vi "S7COMM - Siemens Date & Time to Timestamp.vi"(8 "error in (no error)":errorcluster, 11 "S7 DATE_AND_TIME":u8[](array[numeric])) -> (0 "error out":errorcluster, 1 "Invalid Timestamp":bool, 2 "DT":T1 {"Weekday" items=["Sunday"=1, "Monday"=2, "Tuesday"=3, "Wednesday"=4, "Thursday"=5, "Friday"=6, "Saturday"=7]; "Month" items=["Jan"=1, "Feb"=2, "Mar"=3, "Apr"=4, "May"=5, "Jun"=6, "Jul"=7, "Aug"=8, "Sep"=9, "Oct"=10, "Nov"=11, "Dec"=12]}, 3 "Time Stamp":timestamp)   [LabVIEW 2014, in "S7NetCom.lvclass"]
uses:
  S7NetCom.lvclass
  S7COMM - DTL--cluster.ctl
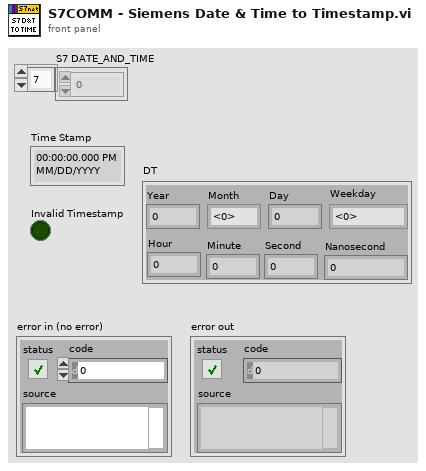
[diagram p1: front panel]
types:
  T1 = typedef "S7NetCom.lvclass/S7COMM - DTL--cluster.ctl" = cluster{"Year":u16, "Month":u8, "Day":u8, "Hour":u8, "Minute":u8, "Second":u8, "Nanosecond":u32, "Weekday":u8}
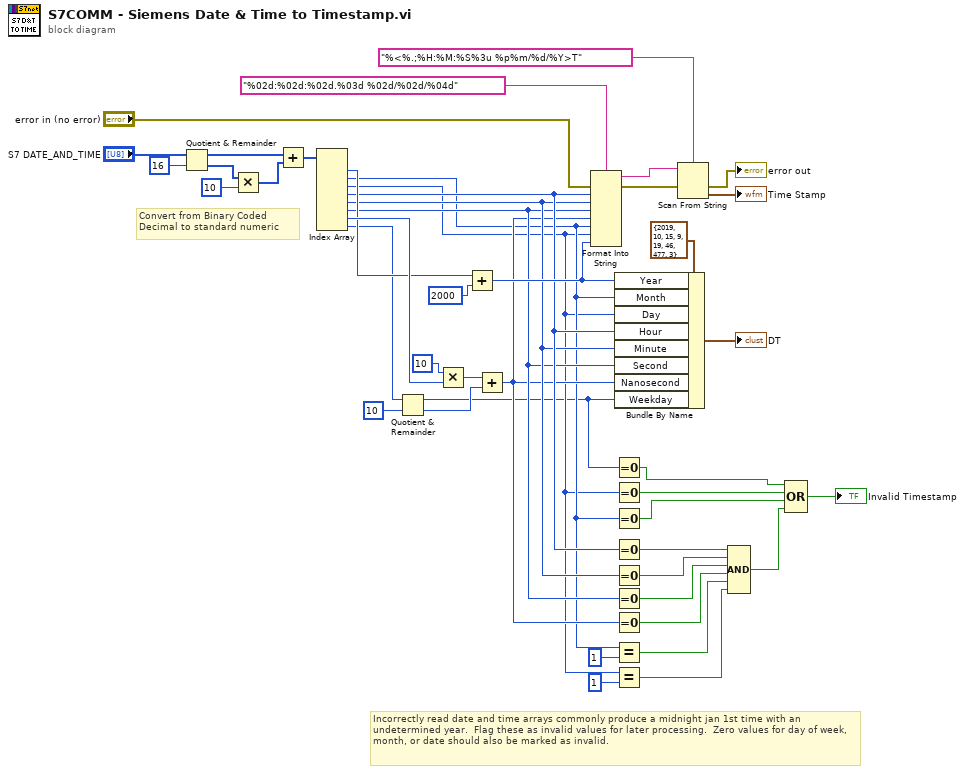
[diagram p0: block diagram]
diagram:
  # "Convert from Binary Coded Decimal to standard numeric"
  # "Incorrectly read date and time arrays commonly produce a midnight jan 1st time with an undetermined year.  Flag these as invalid values for later processing.  Zero values for day of week, month, or date should also be marked as invalid."
  n1 = Quotient & Remainder(x="S7 DATE_AND_TIME", y=u8 16) -> (x-y*floor(x/y)=w4:u8[], floor(x/y)=w2:u8[])
  n2 = Multiply(x=w2, y=u8 10) -> (x*y=w3:u8[])
  n3 = Add(x=w4, y=w3) -> (x+y=w6:u8[])
  n4 = Index Array(array=w6) -> (element #1=w41:u8, element #2=w16:u8, element #3=w15:u8, element #4=w24:u8, element #5=w23:u8, element #6=w22:u8, element #7=w43:u8, element #8=w32:u8)  [unwired: 8 in]
  n5 = Quotient & Remainder(x=w32, y=u8 10) -> (x-y*floor(x/y)=w9:u8, floor(x/y)=w30:u8)
  n6 = Multiply(x=u32 10, y=w43) -> (x*y=w45:u32)
  n7 = Add(x=w41, y=2000 ("x")) -> (x+y=w34:i32)
  n8 = Add(x=w45, y=w30) -> (x+y=w21:u32)
  n9 = Format Into String(format string="%02d:%02d:%02d.%03d %02d/%02d/%04d", error in="error in (no error)", w24, w23, w22, w21, w16, w15, w34) -> (resulting string=w39:string, error out=w28:errorcluster)  [unwired: 1 in]
  n10 = Equal To 0?(x=w9) -> (x = 0?=w8:bool)
  n11 = Equal To 0?(x=w15) -> (x = 0?=w27:bool)
  n12 = Equal To 0?(x=w16) -> (x = 0?=w25:bool)
  n13 = Equal To 0?(x=w24) -> (x = 0?=w20:bool)
  n14 = Equal To 0?(x=w23) -> (x = 0?=w19:bool)
  n15 = Equal To 0?(x=w22) -> (x = 0?=w18:bool)
  n16 = Equal To 0?(x=w21) -> (x = 0?=w17:bool)
  n17 = Equal?(x=w16, y=u8 1) -> (x = y?=w12:bool)
  n18 = Equal?(x=w15, y=u8 1) -> (x = y?=w11:bool)
  n19 = Bundle By Name(cluster=T1 {"Year"=2019, "Month"=10, "Day"=15, "Hour"=9, "Minute"=19, "Second"=46, "Nanosecond"=477, "Weekday"=3} ("DT"), "Year"=w34, "Month"=w16, "Day"=w15, "Hour"=w24, "Minute"=w23, "Second"=w22, "Nanosecond"=w21, "Weekday"=w9) -> (→"DT":T1)
  n20 = Scan From String(format string="%<%.;%H:%M:%S%3u %p%m/%d/%Y>T", input string=w39, error in=w28) -> (error out=→"error out":errorcluster, output 1=→"Time Stamp":timestamp)  [unwired: 2 in, 2 out]
  n21 = Compound Arithmetic op=AND(w20, w19, w18, w17, w12, w11) -> (w10:bool)
  n22 = Compound Arithmetic op=OR(w8, w27, w25, w10) -> (→"Invalid Timestamp":bool)
